vi "Case_Structure.vi"() -> ()   [LabVIEW 2022 SP3]
panel:
  out "String":string
  in  "Boolean":bool
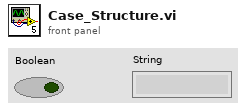
[diagram p1: front panel]
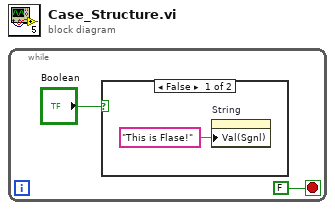
[diagram p0: block diagram]
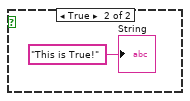
[diagram p2: hidden frame]
diagram:
  n1 = while {
    stop <- FALSE stop-if-true
    n2 = case shown="False" "Boolean" {
      frame False {
        n3 = property on="String" class="Str"("Val(Sgnl)"="This is Flase!" ("Value (Signaling)")) -> ()  [unwired: 2 in, 2 out]
      }
      frame True {
        "String" <- "This is True!" ("String")
      }
    }
  }
